vi "example_simple_qa.vi"() -> ()   [LabVIEW 2020]
uses:
  src/models/llm_openai_chatmodels/llm_openai_chatmodels.lvclass
  D:/Personal/LabVIEW LLMs/src/models/abstract_llm_base/abstract_llm_base.lvclass
  src/vectorstore/vector_qdrant/vector_qdrant.lvclass
  D:/Personal/LabVIEW LLMs/src/vectorstore/abstract_vector_base/abstract_vector_base.lvclass
  src/models/llm_openai_embedding/llm_openai_embedding.lvclass
  src/models/message_text/message_text.lvclass
  D:/Personal/LabVIEW LLMs/src/models/abstract_message_base/abstract_message_base.lvclass
  src/models/llm_openai_chatmodels/Instantiate_llm_openai.vi
  src/models/llm_openai_embedding/Instantiate_llm_openai_embed.vi
  src/models/message_text/get_text_message_value.vi
  src/models/message_text/create_text_message.vi
  src/models/abstract_message_base/abstract_message_base.lvclass
  src/agent/agent_simple_qa/agent_simple_qa.lvclass
  src/utilities/env_variables/env_variables.lvlib
panel:
  in  "send":bool
  in  "new_message":string
  out "Messages":cluster{"role":string, "text":string}[](array[cluster])
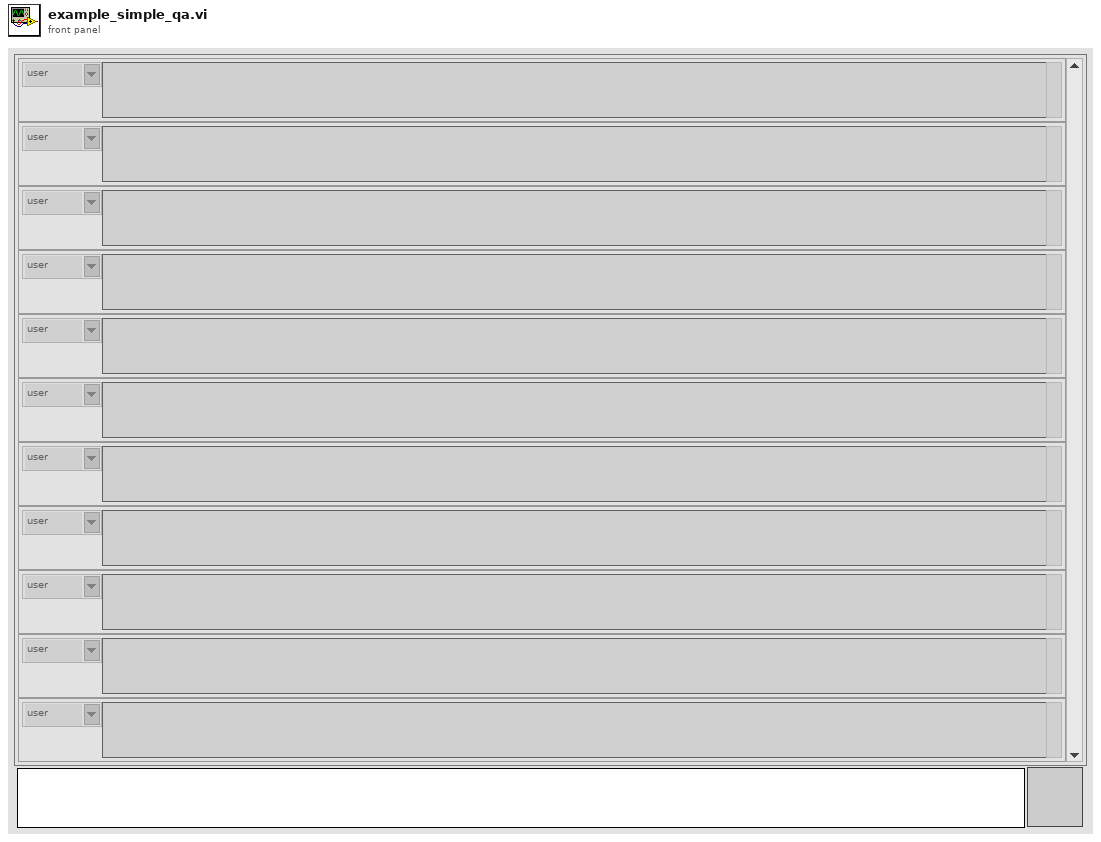
[diagram p1: front panel]
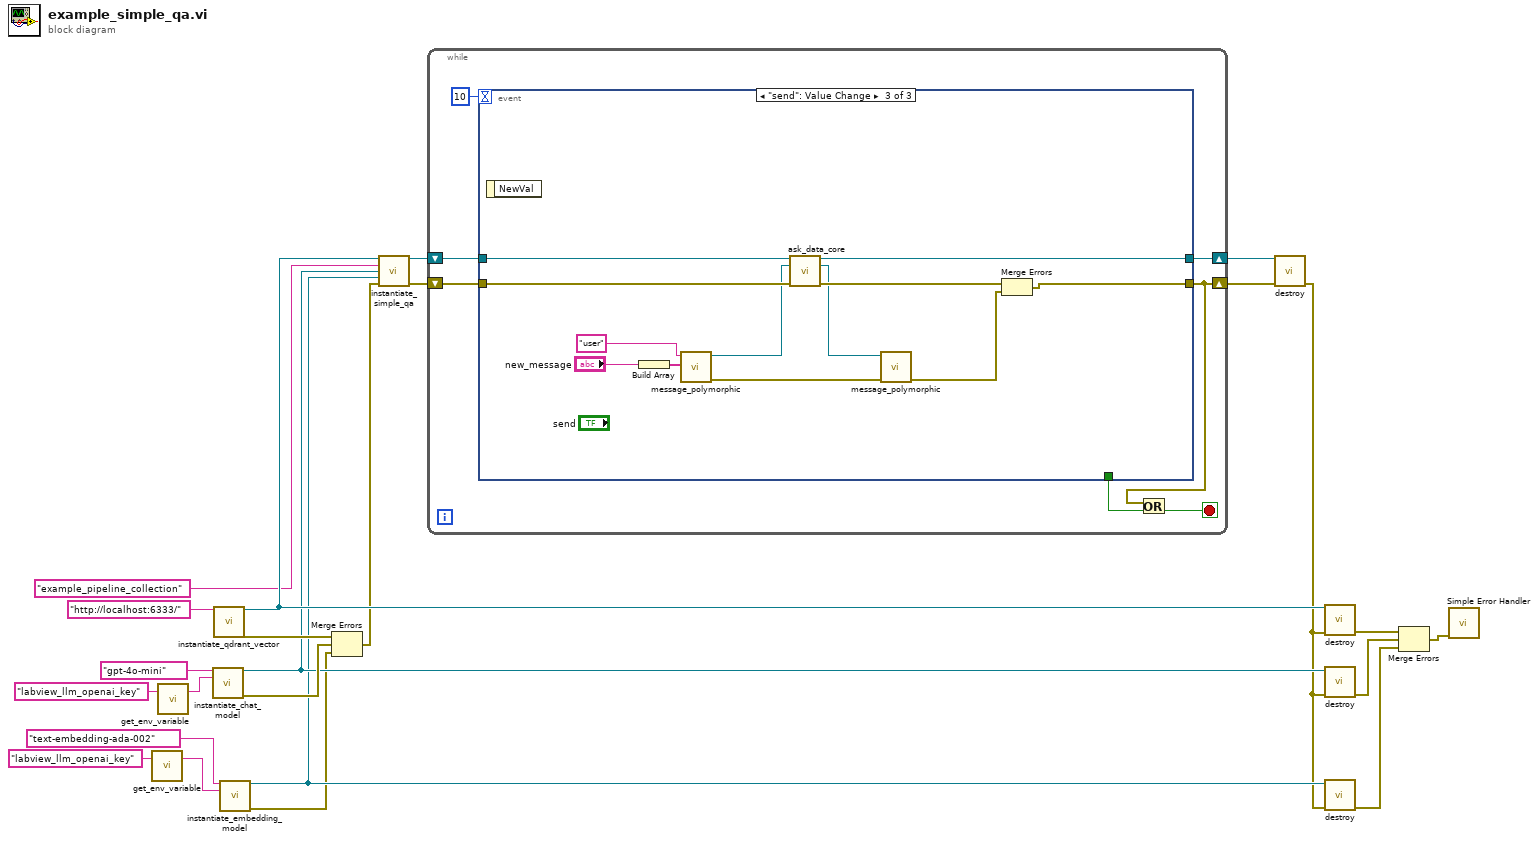
[diagram p0: block diagram]
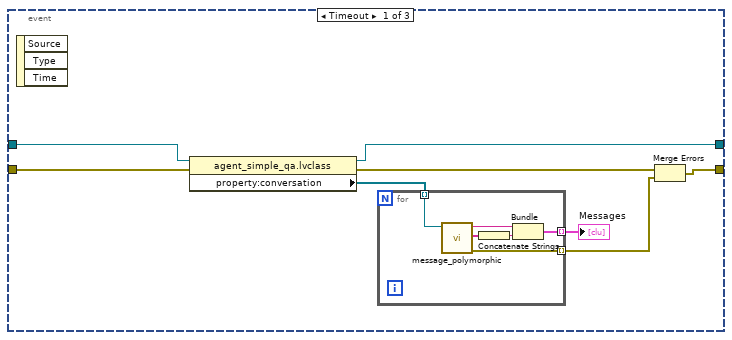
[diagram p2: hidden frame]
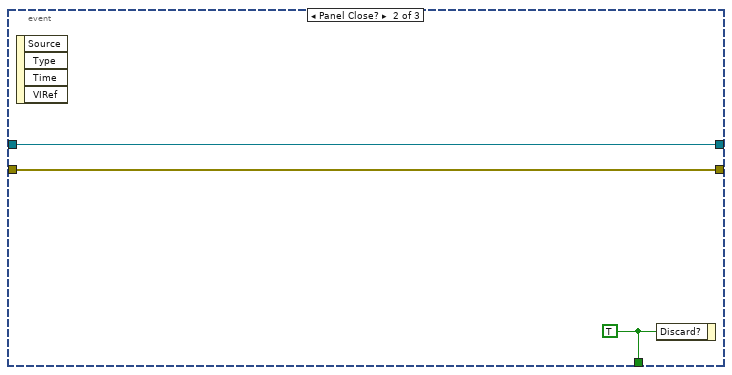
[diagram p3: hidden frame]
diagram:
  n1 = call "get_env_variable.vi"("Environment Variable Name"="labview_llm_openai_key") -> ("Value"=w5:string)  [unwired: 1 in, 1 out]
  n2 = call "get_env_variable.vi"("Environment Variable Name"="labview_llm_openai_key") -> ("Value"=w18:string)  [unwired: 1 in, 1 out]
  n3 = call-poly "instantiate_chat_model.vi"("model_name"="gpt-4o-mini", "openai_key"=w18) -> ("llm_openai out"=w9:refnum<class "llm_openai_chatmodels.lvclass">, "error out"=w11:errorcluster)  [unwired: 12 in]
  n4 = call "instantiate_qdrant_vector.vi"("host_url"="http://localhost:6333/") -> ("vector_qdrant out"=w16:refnum<class "vector_qdrant.lvclass">, "error out"=w12:errorcluster)  [unwired: 13 in]
  n5 = call-poly "instantiate_embedding_model.vi"("model_name"="text-embedding-ada-002", "openai_key"=w5) -> ("llm_openai_embedding out"=w4:refnum<class "llm_openai_embedding.lvclass">, "error out"=w3:errorcluster)  [unwired: 12 in]
  n6 = Merge Errors(w12, w11, w3) -> (w10:errorcluster)
  n7 = call "instantiate_simple_qa.vi"("vectorestore"=w16, "collection_name"="example_pipeline_collection" ("host_url"), "chat_model"=w9, "embedding_model"=w4, "error in (no error)"=w10) -> ("agent_simple_qa out"=w24:refnum<class "agent_simple_qa.lvclass">, "error out"=w23:errorcluster)  [unwired: 9 in]
  n8 = while {
    shift-right: [w28] -> w22
    shift-left: w24 -> [w29]
    shift-right: [w25] -> w21
    shift-left: w23 -> [w27]
    stop <- w26 stop-if-true
    n9 = event shown="[2] \"send\": Value Change" {
      selector: _ -> [_ _ _]
      dyn-events: _ -> [_ _ _]
      timeout: 10 -> [_ _ _]
      tunnel: [_ w48 _] -> w31
      tunnel: w29 -> [w38 w47 w60]
      tunnel: [w36 w47 w59] -> w28
      tunnel: w27 -> [w39 w46 w58]
      tunnel: [w33 w46 w50] -> w25
      event Timeout {
        n10 = event-data() -> ()  [unwired: 1 in, 3 out]
        n11 = property class="agent_simple_qa.lvclass"(reference=w38, error in=w39) -> (reference out=w36:refnum<class "agent_simple_qa.lvclass">, error out=w37:errorcluster, "property:conversation"=w35:refnum<class "abstract_message_base.lvclass">[])
        n12 = for {
          tunnel: w35 -> [w45] mode=indexing
          tunnel: [w41] -> w34 mode=indexing
          tunnel: [w40] -> w32 mode=indexing
          n13 = call-poly "message_polymorphic.vi"("abstract_message_base.lvclass"=w45) -> ("error out"=w40:errorcluster, "content"=w43:string[], "role"=w44:string)  [unwired: 8 in]
          n14 = Concatenate Strings(w43) -> (w42:string)
          n15 = Bundle("role"=w44, w42) -> (w41:cluster{"role":string, string})  [unwired: 1 in]
        }
        "Messages" <- w34
        n16 = Merge Errors(w37, w32) -> (w33:errorcluster)
      }
      event Panel Close? {
        w48 = TRUE ("Discard?")
        n17 = event-data() -> ()  [unwired: 1 in, 4 out]
        n18 = event-data("Discard?"=w48) -> ()  [unwired: 1 in, 1 out]
      }
      event "send": Value Change {
        n19 = event-data() -> ()  [unwired: 1 in, 1 out]
        n20 = Build Array("new_message") -> (w54:string[])
        n21 = call-poly "message_polymorphic.vi"("content"=w54, "role"="user") -> ("error out"=w51:errorcluster, "message_text out"=w53:refnum<class "message_text.lvclass">)  [unwired: 8 in]
        n22 = call-dynamic "ask_data_core.vi"("agent_simple_qa in"=w60, "message"=w53, "error in (no error)"=w58) -> ("agent_simple_qa out"=w59:refnum<class "agent_simple_qa.lvclass">, "assisstant_response"=w52:refnum<class "abstract_message_base.lvclass">, "error out"=w57:errorcluster)  [unwired: 10 in]
        n23 = call-poly "message_polymorphic.vi"("error in"=w51, "abstract_message_base.lvclass"=w52) -> ("error out"=w49:errorcluster)  [unwired: 7 in, 2 out]
        n24 = Merge Errors(w57, w49) -> (w50:errorcluster)
      }
    }
    n25 = Or(x=w25, y=w31) -> (x .or. y?=w26:bool)
  }
  n26 = call-dynamic "destroy.vi"("agent_simple_qa in"=w22, "error in (no error)"=w21) -> ("error out"=w2:errorcluster)  [unwired: 12 in, 1 out]
  n27 = call-dynamic "destroy.vi"("vector_qdrant in"=w16, "error in (no error)"=w2) -> ("error out"=w15:errorcluster)  [unwired: 12 in, 1 out]
  n28 = call-dynamic "destroy.vi"("error in (no error)"=w2, "abstract_llm_base in"=w9) -> ("error out"=w14:errorcluster)  [unwired: 8 in, 1 out]
  n29 = call-dynamic "destroy.vi"("error in (no error)"=w2, "llm_openai_embedding in"=w4) -> ("error out"=w1:errorcluster)  [unwired: 8 in, 1 out]
  n30 = Merge Errors(w15, w14, w1) -> (w13:errorcluster)
  n31 = call <vilib>:"Simple Error Handler.vi"("error in (no error)"=w13) -> ()  [unwired: 4 in, 5 out]
